vi "QX_Search QX Devices.vi"(8 "error in":errorcluster) -> (0 "error out":errorcluster, 2 "QX DevInfo":T1[](array[typedef]), 3 "Devices":refnum<k24>[](array[refnum]))   [LabVIEW 2016]
uses:
  QX Module Info.ctl
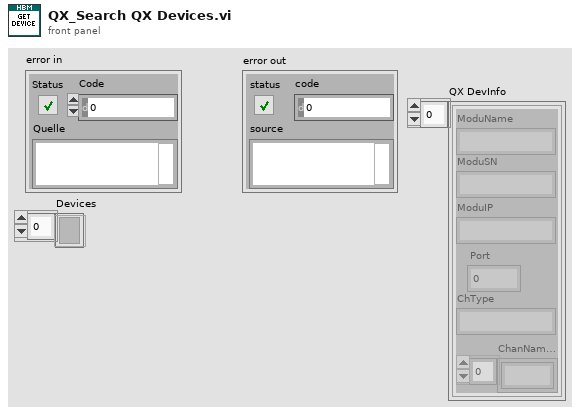
[diagram p1: front panel]
types:
  T1 = typedef "QX Module Info.ctl" = cluster{"ModuName":string, "ModuSN":string, "ModuIP":string, "Port":i32, "ChType":string, "ChanNames[]":string[]}
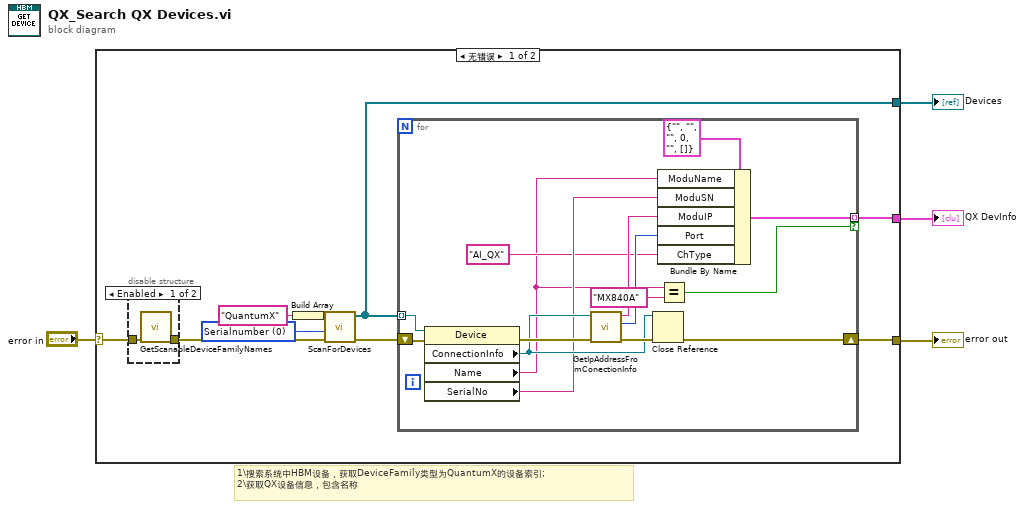
[diagram p0: block diagram]
diagram:
  # "1\\搜索系统中HBM设备，获取DeviceFamily类型为QuantumX的设备索引;\n2\\获取QX设备信息，包含名称"
  n1 = case shown="无错误" "error in" {
    selector: "error in" -> [w6 w32]
    tunnel: [w13 w32] -> w3
    tunnel: [w12 _] -> w2
    tunnel: [w5 _] -> w1
    frame No Error {
      w10 = 0 items=["Serialnumber", "Name", "IpAddress"] ("SortedBy")
      n2 = disable-structure shown="Enabled" {
        disable-tunnel: w6 -> [w30 w31]
        disable-tunnel: [w29 w31] -> w9
        frame Enabled {
          n3 = call "GetScanableDeviceFamilyNames.vi"("Error in"=w30) -> ("Error out"=w29:errorcluster)  [unwired: 8 in, 2 out]
        }
        frame Disabled {
        }
      }
      n4 = Build Array("QuantumX") -> (w11:string[])
      n5 = call "ScanForDevices.vi"("Error in"=w9, "SortedBy"=w10, "AvailableDeviceFamilies"=w11) -> ("Error out"=w8:errorcluster, "Devices"=w12:refnum<k24>[])  [unwired: 7 in]
      n6 = for {
        tunnel: w12 -> [w28] mode=indexing
        shift-right: [w24] -> w13
        shift-left: w8 -> [w27]
        tunnel: [w19] -> w5 mode=indexing if=w14
        n7 = property class="Device"(reference=w28, error in=w27) -> (error out=w26:errorcluster, "ConnectionInfo"=w23:refnum<k24>, "Name"=w16:string, "SerialNo"=w20:string)  [unwired: 1 out]
        n8 = call "GetIpAddressFromConectionInfo.vi"("Error in"=w26, "ConnectionInfo"=w23) -> ("Error out"=w25:errorcluster, "Port"=w18:i32, "IpAddress"=w21:string)  [unwired: 7 in]
        n9 = Close Reference(reference=w23, error in (no error)=w25) -> (error out=w24:errorcluster)
        n10 = Bundle By Name(cluster=T1 {"ModuName"="", "ModuSN"="", "ModuIP"="", "Port"=0, "ChType"="", "ChanNames[]"=[]} ("DevInfo"), "ModuName"=w16, "ModuSN"=w20, "ModuIP"=w21, "Port"=w18, "ChType"="AI_QX") -> (w19:T1)
        n11 = Equal?(x=w16, y="MX840A") -> (x = y?=w14:bool)
      }
    }
    frame Error {
    }
  }
  "error out" <- w3
  "Devices" <- w2
  "QX DevInfo" <- w1
